vi "MakePlot.vi"(5 "Polarity array":refnum<vi>[](array[refnum]), 6 "Amplitude array":refnum<vi>[](array[refnum]), 7 "Channel array":refnum<vi>[](array[refnum])) -> (0 "min value":dbl, 1 "Numeric 3":dbl, 2 "samples":i32, 3 "Numeric":T1 min=-999.0 max=999.0 format="%+.12f", 4 "Array":cluster{"Pulse Pattern":dbl[]}[](array[cluster]))   [LabVIEW 2020]
uses:
  DelayControl2.ctl
  <vilib>/Analysis/NI_AALBase.lvlib
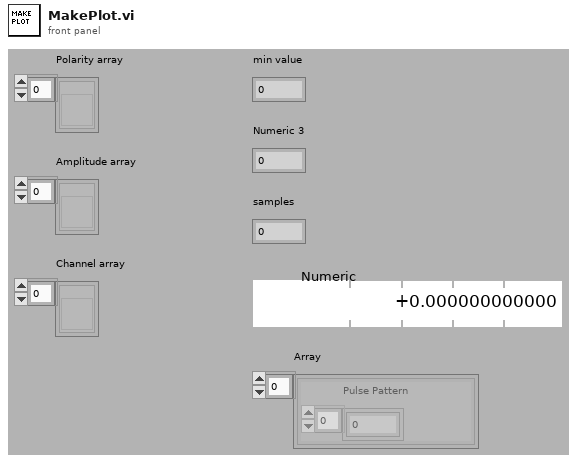
[diagram p1: front panel]
types:
  T1 = typedef "DelayControl2.ctl" = dbl
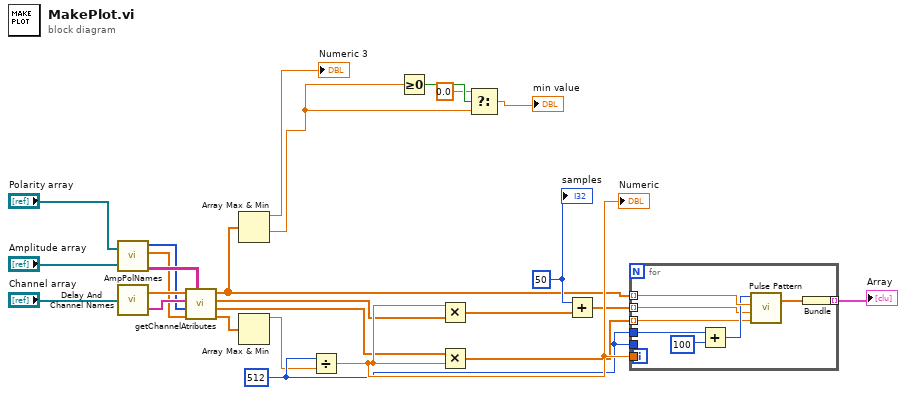
[diagram p0: block diagram]
diagram:
  w21 = 50 ("samples")
  w20 = 512 ("samples")
  n1 = call "AmpPolNames.vi"("Polarity array"="Polarity array", "Amplitude array"="Amplitude array") -> ("Array 2"=w8:enum16{"Negative", "Positive"}[], "Array 3"=w7:dbl[], "Array"=w9:string[][])  [unwired: 1 out]
  n2 = call "Delay And Channel Names.vi"("Channel array"="Channel array") -> ("Array"=w11:T1[], "Array 2"=w10:string[])
  n3 = call "getChannelAtributes.vi"("Ch Name 2"=w9, "amplitude"=w7, "polarity"=w8, "Ch Name"=w10, "Delay"=w11) -> ("Array 4"=w13:T1[], "Array 2"=w15:T1[], "Array"=w17:T1[], "Array 3"=w14:dbl[])  [unwired: 1 in]
  n4 = Array Max & Min(array=w14) -> (max value=→"Numeric 3":dbl, min value=w2:dbl)  [unwired: 2 out]
  n5 = Array Max & Min(array=w13) -> (max value=w12:T1)  [unwired: 3 out]
  n6 = Divide(x=w20, y=w12) -> (x/y=w22:T1)
  "Numeric" <- w22
  n7 = Greater Or Equal To 0?(x=w2) -> (x >= 0?=w4:bool)
  n8 = Multiply(x=w22, y=w17) -> (x*y=w18:T1[])
  n9 = Multiply(x=w15, y=w22) -> (x*y=w16:T1[])
  n10 = Select(t=0.0, s=w4, f=w2) -> (s? t:f=→"min value":dbl)
  n11 = Add(x=w21, y=w18) -> (x+y=w19:T1[])
  n12 = for {
    tunnel: w20 -> [_]
    tunnel: w14 -> [w33] mode=indexing
    tunnel: w16 -> [w28] mode=indexing
    tunnel: [w31] -> w25 mode=indexing
    tunnel: w22 -> [_]
    tunnel: w19 -> [w27] mode=indexing
    tunnel: w20 -> [w26]
    n13 = Add(x=w26, y=100) -> (x+y=w30:i32)
    n14 = call <vilib>:"Pulse Pattern.vi"("width"=w28, "delay"=w27, "amplitude"=w33, "samples"=w30) -> ("Pulse Pattern"=w32:dbl[])  [unwired: 1 out]
    n15 = Bundle("Pulse Pattern"=w32) -> (w31:cluster{"Pulse Pattern":dbl[]})  [unwired: 1 in]
  }
  "Array" <- w25
  "samples" <- w21
